vi "DIO write.vi"(8 "error in (no error)":errorcluster, 10 "output":bool, 11 "DIO in":refnum<class "DIO.lvclass">) -> (0 "error out":errorcluster, 3 "DIO out":refnum<class "DIO.lvclass">)   [LabVIEW 2019, in "my FPGA lib.lvlib" / "DIO.lvclass"]
uses:
  DIO.lvclass
  DIO.lvclass/DIO.ctl
  <vilib>/Utility/error.llb/Error Cluster From Error Code.vi
  <vilib>/rvi/errors/niLvFpgaAdjustHostInterfaceError.vi
  <vilib>/rvi/interface/nirviReadWriteControl/nirviReadWriteControl.xnode
  NiFpgaLv.dll
  <vilib>/rvi/interface/Simulation/niFpgaSimulationCallBeginRW.vi
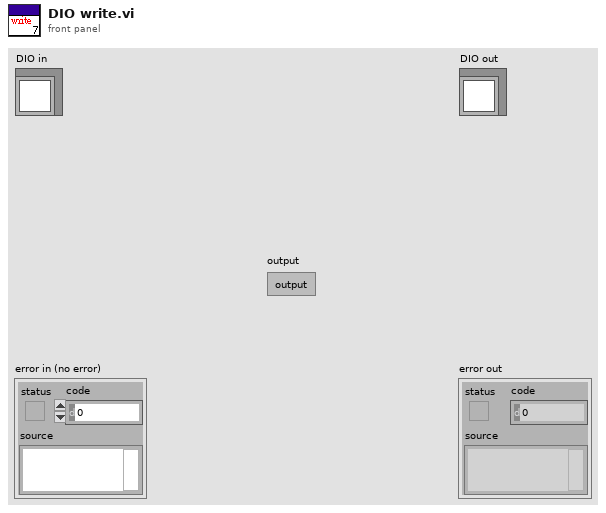
[diagram p1: front panel]
types:
  T1 = typedef "my FPGA lib.lvlib/DIO.lvclass/DIO enum.ctl" = enum16{"US.1", "US.2", "US.3", "US.4", "C.0", "C.1", "C.2", "C.3", "C.4", "C.5", "C.6", "C.7", "B.14", "B.15"}
  T2 = typedef "my FPGA lib.lvlib/DIO.lvclass/port.ctl" = enum16{"US", "C.", "B."}
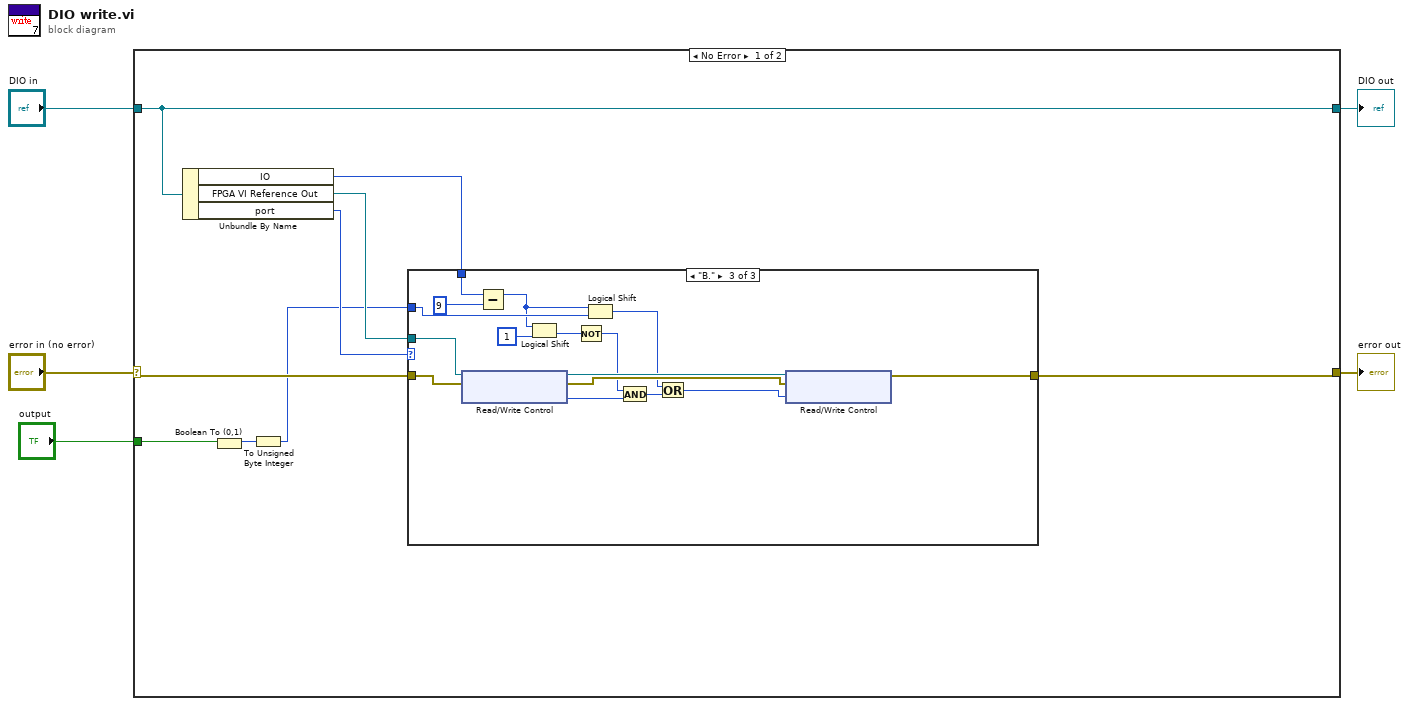
[diagram p0: block diagram]
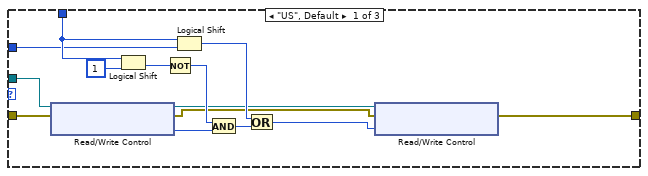
[diagram p2: hidden frame]
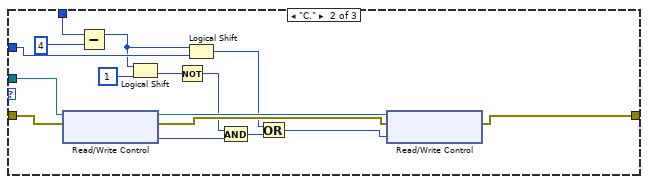
[diagram p3: hidden frame]
diagram:
  n1 = case shown="No Error" "error in (no error)" {
    selector: "error in (no error)" -> [w11 w62]
    tunnel: [w6 w62] -> w4
    tunnel: [w14 w61] -> w2
    tunnel: "DIO in" -> [w14 w61]
    tunnel: "output" -> [w9 _]
    frame No Error {
      n2 = Unbundle By Name(w14) -> ("IO"=w10:T1, "FPGA VI Reference Out"=w12:refnum<k20>, "port"=w13:T2)
      n3 = Boolean To (0,1)(Boolean=w9) -> (0, 1=w8:i16)
      n4 = To Unsigned Byte Integer(number=w8) -> (unsigned 8bit integer=w7:u8)
      n5 = case shown="\"B.\"" w13 {
        tunnel: w12 -> [w28 w32 w48]
        tunnel: w11 -> [w27 w33 w49]
        tunnel: w10 -> [w22 w35 w51]
        tunnel: w7 -> [w21 w34 w50]
        tunnel: [w15 w31 w47] -> w6
        frame "US", Default {
          n6 = xnode "Read/Write Control"("FPGA VI Reference In"=w28, "error in"=w27) -> ("FPGA VI Reference Out"=w17:refnum<k20>, "error out"=w16:errorcluster, "Ultrasonic.IO.Write"=w23:u8)
          n7 = Logical Shift(y=w22, x=u8 1) -> (x << y=w25:u8)
          n8 = Not(x=w25) -> (.not. x?=w24:u8)
          n9 = Logical Shift(y=w22, x=w21) -> (x << y=w19:u8)
          n10 = And(x=w24, y=w23) -> (x .and. y?=w20:u8)
          n11 = Or(x=w19, y=w20) -> (x .or. y?=w18:u8)
          n12 = xnode "Read/Write Control"("FPGA VI Reference In"=w17, "error in"=w16, "Ultrasonic.IO.Write"=w18) -> ("error out"=w15:errorcluster)  [unwired: 1 out]
        }
        frame "C." {
          n13 = xnode "Read/Write Control"("FPGA VI Reference In"=w32, "error in"=w33) -> ("FPGA VI Reference Out"=w43:refnum<k20>, "error out"=w44:errorcluster, "Basic IO Write"=w39:u8)
          n14 = Subtract(x=w35, y=4) -> (x-y=w30:i32)
          n15 = Logical Shift(y=w30, x=u8 1) -> (x << y=w37:u8)
          n16 = Not(x=w37) -> (.not. x?=w38:u8)
          n17 = Logical Shift(y=w30, x=w34) -> (x << y=w41:u8)
          n18 = And(x=w38, y=w39) -> (x .and. y?=w40:u8)
          n19 = Or(x=w41, y=w40) -> (x .or. y?=w42:u8)
          n20 = xnode "Read/Write Control"("FPGA VI Reference In"=w43, "error in"=w44, "Basic IO Write"=w42) -> ("error out"=w31:errorcluster)  [unwired: 1 out]
        }
        frame "B." {
          n21 = xnode "Read/Write Control"("FPGA VI Reference In"=w48, "error in"=w49) -> ("FPGA VI Reference Out"=w59:refnum<k20>, "error out"=w60:errorcluster, "Basic.2 IO Write"=w55:u8)
          n22 = Subtract(x=w51, y=9) -> (x-y=w46:i32)
          n23 = Logical Shift(y=w46, x=u8 1) -> (x << y=w53:u8)
          n24 = Not(x=w53) -> (.not. x?=w54:u8)
          n25 = Logical Shift(y=w46, x=w50) -> (x << y=w57:u8)
          n26 = And(x=w54, y=w55) -> (x .and. y?=w56:u8)
          n27 = Or(x=w57, y=w56) -> (x .or. y?=w58:u8)
          n28 = xnode "Read/Write Control"("FPGA VI Reference In"=w59, "error in"=w60, "Basic.2 IO Write"=w58) -> ("error out"=w47:errorcluster)  [unwired: 1 out]
        }
      }
    }
    frame Error {
    }
  }
  "error out" <- w4
  "DIO out" <- w2
